vi "Initialize Data.vi"(8 "error in (no error)":errorcluster, 9 "data version":T1, 10 "data":string, 11 "Core Transfers Configuration in":refnum<class "Core Transfers Configuration.lvclass">) -> (0 "error out":errorcluster, 3 "Core Transfers Configuration out":refnum<class "Core Transfers Configuration.lvclass">)   [LabVIEW 2017, in "DSF Core.lvlib" / "Core Transfers Configuration.lvclass"]
uses:
  Core Transfers Configuration.lvclass
  Typedefs/DSF Version Info.ctl
  Core Transfers Configuration.lvclass/Core Transfers Configuration.ctl
  DSF Core.lvlib
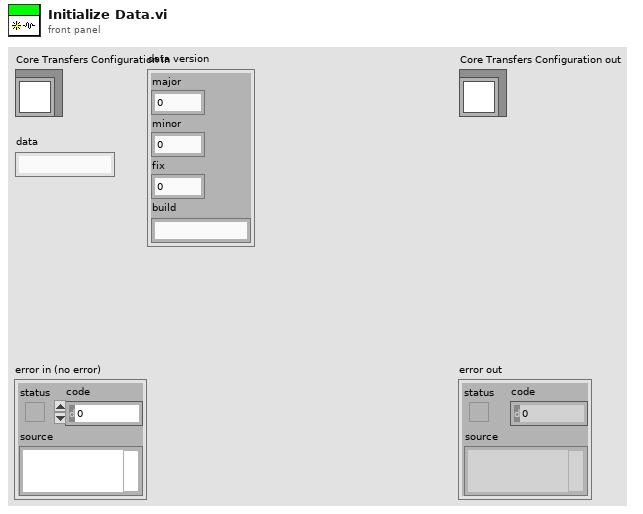
[diagram p1: front panel]
types:
  T1 = typedef "DSF Core.lvlib/DSF Version Info.ctl" = cluster{"major":i32, "minor":i32, "fix":i32, "build":string}
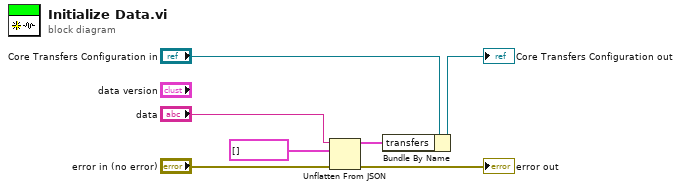
[diagram p0: block diagram]
diagram:
  n1 = Unflatten From JSON(JSON string="data", type and defaults=cluster{"name":string}[] [] ("transfers"), error in (no error)="error in (no error)") -> (value=w2:cluster{"name":string}[], error out=→"error out":errorcluster)  [unwired: 4 in]
  n2 = Bundle By Name(cluster="Core Transfers Configuration in", "transfers"=w2) -> (→"Core Transfers Configuration out":refnum<class "Core Transfers Configuration.lvclass">)
